vi "SubVi-结果计算-从-已知kb求xy.vi"(9 "X-B":dbl, 10 "X-K":dbl, 11 "X value In":dbl) -> (3 "X value Out":dbl)   [LabVIEW 2015]
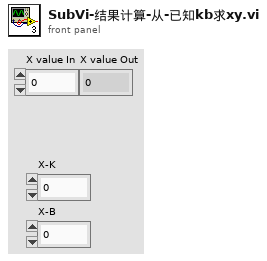
[diagram p1: front panel]
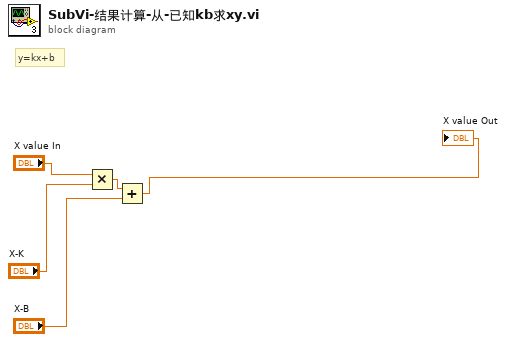
[diagram p0: block diagram]
diagram:
  # "y=kx+b"
  n1 = Multiply(x="X value In", y="X-K") -> (x*y=w3:dbl)
  n2 = Add(x=w3, y="X-B") -> (x+y=→"X value Out":dbl)
